vi "TA.vi"(0 "Folder Name":string, 1 "Name of File":string, 2 "Folder to Save":path, 3 "Timepoints":dbl[](array[numeric]), 4 "Vx array":dbl[](array[numeric]), 5 "Vy array":dbl[](array[numeric])) -> ()   [LabVIEW 2014]
uses:
  <vilib>/Utility/file.llb/Write Delimited Spreadsheet (DBL).vi
  <vilib>/Utility/file.llb/Read Delimited Spreadsheet (DBL).vi
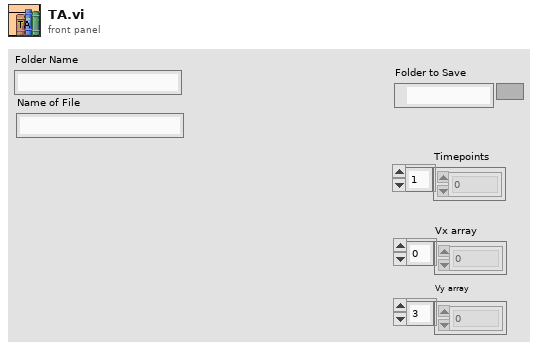
[diagram p1: front panel]
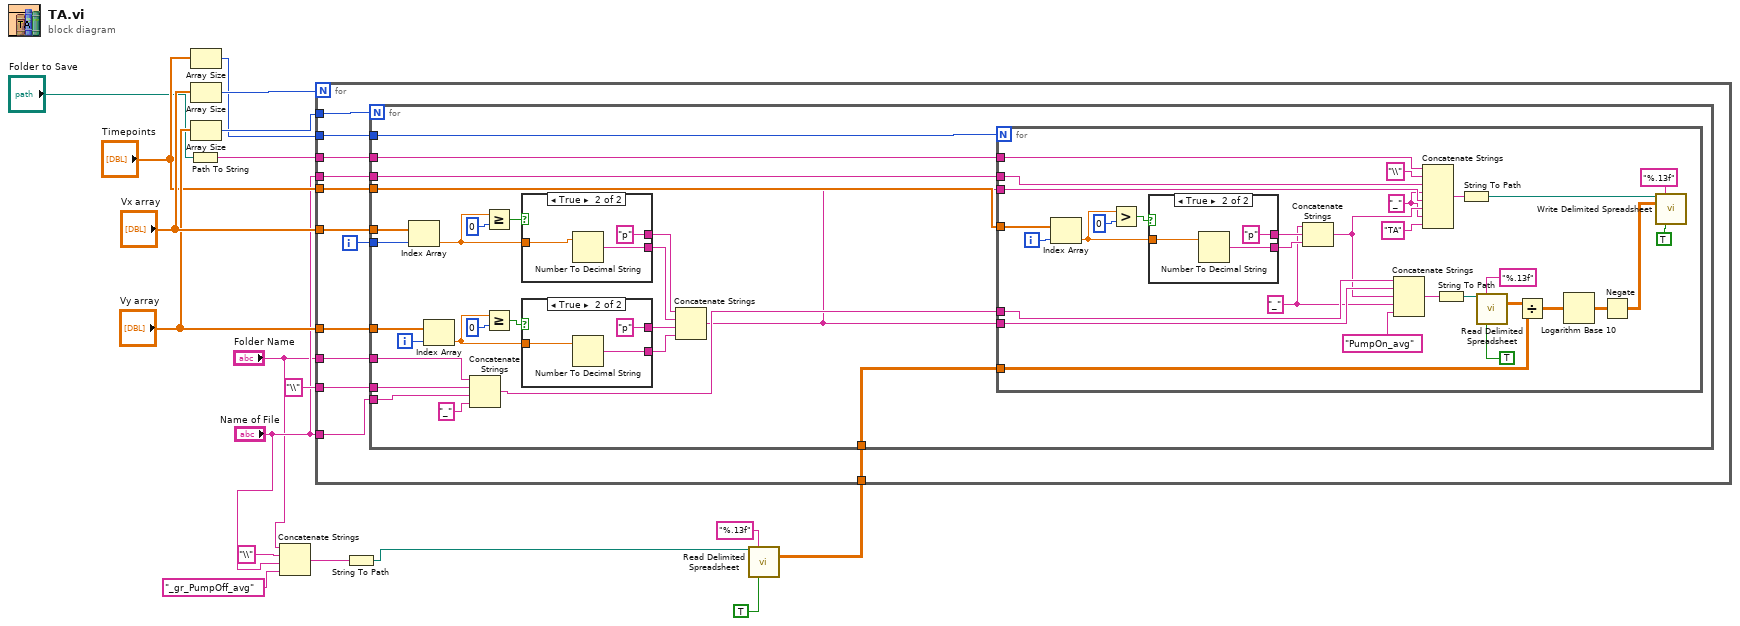
[diagram p0: block diagram]
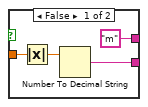
[diagram p2: hidden frame]
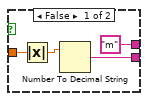
[diagram p3: hidden frame]
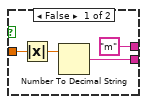
[diagram p4: hidden frame]
diagram:
  n1 = Path To String(path="Folder to Save") -> (string=w11:string)
  n2 = Array Size(array="Timepoints") -> (size(s)=w15:i32)
  n3 = Array Size(array="Vx array") -> (size(s)=w17:i32)
  n4 = Array Size(array="Vy array") -> (size(s)=w16:i32)
  n5 = Concatenate Strings("Folder Name", "\\" ("string"), "Name of File", "_gr_PumpOff_avg" ("string")) -> (w3:string)
  n6 = String To Path(string=w3) -> (path=w2:path)
  n7 = call-poly <vilib>:"Read Delimited Spreadsheet.vi"("file path (dialog if empty)"=w2, "format (%.3f)"="%.13f", "transpose? (F)"=TRUE) -> ("all rows"=w8:dbl[][])  [unwired: 7 in, 5 out]
  n8 = for {
    N: w17 -> [_]
    tunnel: "Name of File" -> [w30]
    tunnel: "\\" -> [w29]
    tunnel: "Folder Name" -> [w28]
    tunnel: w16 -> [w27]
    tunnel: w15 -> [w26]
    tunnel: "Vx array" -> [w25]
    tunnel: "Vy array" -> [w23]
    tunnel: "Timepoints" -> [w22]
    tunnel: w11 -> [w21]
    tunnel: "Name of File" -> [w20]
    tunnel: w8 -> [w19]
    i -> [w24]
    n9 = for {
      N: w27 -> [_]
      tunnel: w30 -> [w32]
      tunnel: w29 -> [w33]
      tunnel: w28 -> [w55]
      tunnel: w26 -> [w54]
      tunnel: w25 -> [w50]
      tunnel: w24 -> [w51]
      tunnel: w23 -> [w45]
      tunnel: w22 -> [w39]
      tunnel: w21 -> [w38]
      tunnel: w20 -> [w37]
      tunnel: w19 -> [w31]
      i -> [w44]
      n10 = Index Array(array=w50, index=w51) -> (element=w49:dbl)
      n11 = Index Array(array=w45, index=w44) -> (element=w46:dbl)
      n12 = Concatenate Strings(w55, w33, w32, "_") -> (w35:string)
      n13 = Greater Or Equal?(x=w49, y=0) -> (x >= y?=w52:bool)
      n14 = Greater Or Equal?(x=w46, y=0) -> (x >= y?=w48:bool)
      n15 = case shown="True" w52 {
        tunnel: ["m" "p"] -> w43
        tunnel: w49 -> [w65 w67]
        tunnel: [w63 w68] -> w42
        frame False {
          n16 = Absolute Value(x=w65) -> (abs(x)=w64:dbl)
          n17 = Number To Decimal String(number=w64) -> (decimal integer string=w63:string)  [unwired: 1 in]
        }
        frame True {
          n18 = Number To Decimal String(number=w67) -> (decimal integer string=w68:string)  [unwired: 1 in]
        }
      }
      n19 = case shown="True" w48 {
        tunnel: ["m" "p"] -> w41
        tunnel: w46 -> [w58 w60]
        tunnel: [w56 w61] -> w40
        frame False {
          n20 = Absolute Value(x=w58) -> (abs(x)=w57:dbl)
          n21 = Number To Decimal String(number=w57) -> (decimal integer string=w56:string)  [unwired: 1 in]
        }
        frame True {
          n22 = Number To Decimal String(number=w60) -> (decimal integer string=w61:string)  [unwired: 1 in]
        }
      }
      n23 = Concatenate Strings(w43, w42, w41, w40) -> (w34:string)
      n24 = for {
        N: w54 -> [_]
        tunnel: w39 -> [w97]
        tunnel: w38 -> [w92]
        tunnel: w37 -> [w89]
        tunnel: w35 -> [w83]
        tunnel: w34 -> [w82]
        tunnel: w31 -> [w73]
        tunnel: w34 -> [w79]
        i -> [w96]
        w81 = "_"
        w77 = "_" ("string")
        n25 = Index Array(array=w97, index=w96) -> (element=w99:dbl)
        n26 = Greater?(x=w99, y=0) -> (0:w98:bool)
        n27 = case shown="True" w98 {
          tunnel: ["m" "p"] -> w94
          tunnel: w99 -> [w103 w105]
          tunnel: [w101 w106] -> w95
          frame False {
            n28 = Absolute Value(x=w103) -> (abs(x)=w102:dbl)
            n29 = Number To Decimal String(number=w102) -> (decimal integer string=w101:string)  [unwired: 1 in]
          }
          frame True {
            n30 = Number To Decimal String(number=w105) -> (decimal integer string=w106:string)  [unwired: 1 in]
          }
        }
        n31 = Concatenate Strings(w81, w94, w95) -> (w78:string)
        n32 = Concatenate Strings(w83, w82, w78, w81, "PumpOn_avg") -> (w85:string)
        n33 = Concatenate Strings(w92, "\\" ("string"), w89, w77, w79, w78, w77, "TA" ("string")) -> (w75:string)
        n34 = String To Path(string=w85) -> (path=w86:path)
        n35 = String To Path(string=w75) -> (path=w91:path)
        n36 = call-poly <vilib>:"Read Delimited Spreadsheet.vi"("file path (dialog if empty)"=w86, "format (%.3f)"="%.13f", "transpose? (F)"=TRUE) -> ("all rows"=w74:dbl[][])  [unwired: 7 in, 5 out]
        n37 = Divide(x=w74, y=w73) -> (x/y=w72:dbl[][])
        n38 = Logarithm Base 10(1:w72) -> (0:w71:dbl[][])
        n39 = Negate(x=w71) -> (-x=w70:dbl[][])
        n40 = call-poly <vilib>:"Write Delimited Spreadsheet.vi"("file path (dialog if empty)"=w91, "format (%.3f)"="%.13f", "2D data"=w70, "transpose? (F)"=TRUE) -> ()  [unwired: 10 in, 2 out]
      }
    }
  }
